vi "set range property lecroy.vi"(0 "VISA in":refnum<visa-resource-name>, 5 "Group":string, 7 "Property":T1, 9 "Value":variant, 11 "error in":errorcluster, 12 "First Channel":T2={" Card.Channel"=1.12, "Crate"=0} {"Card.Channel" format="%.2f"}, 13 "Num Channels":i32) -> (4 "VISA out":refnum<visa-resource-name>, 15 "error out":errorcluster)   [LabVIEW 2018]
uses:
  channel.ctl
  Group Properties.ctl
  Tom Shaw/Lecroy Control/HV Documentation and Software for Testing/SubVIs/General_lecroy_command.ctl
  CAEN globals.vi
  <vilib>/regexp/Match Regular Expression.xnode
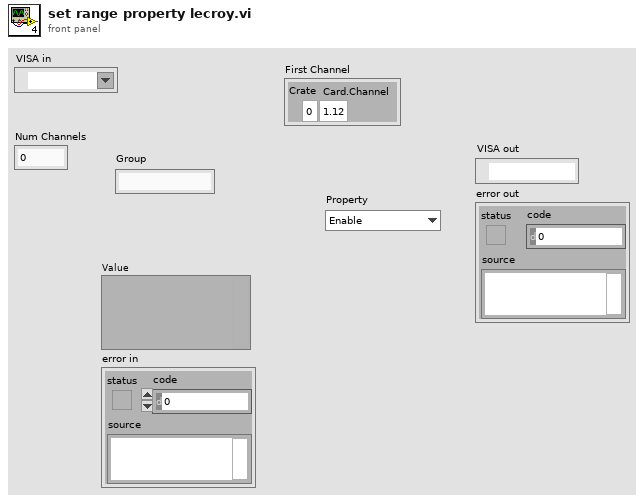
[diagram p1: front panel]
types:
  T1 = typedef "Group Properties.ctl" = enum16{"Enable", "Vset", "Imax", "Vswmax", "Trip Time"}
  T2 = typedef "channel.ctl" = cluster{" Card.Channel":dbl, "Crate":i32}
  T3 = enum16{"Monitor", "Demand", "Backup", "All", "None"}
  T4 = typedef "General_lecroy_command.ctl" = string
  T5 = typedef "channel_cluster.ctl" = cluster{"Channel Name":string, "Crate":i32, "Card Type":string, "Card":i32, "Channel":i32, "Status Icon":picture, "Vmon (V)":dbl, "Vset (V)":dbl, "Imon (A)":dbl, "Iset (A)":dbl, "Timestamp":string, "ON/OFF":bool, "Status":string, "Vswmax (V)":dbl, "Flag":bool, "Vfile (V)":dbl, "Error Logged":bool[], "enable_file":bool}
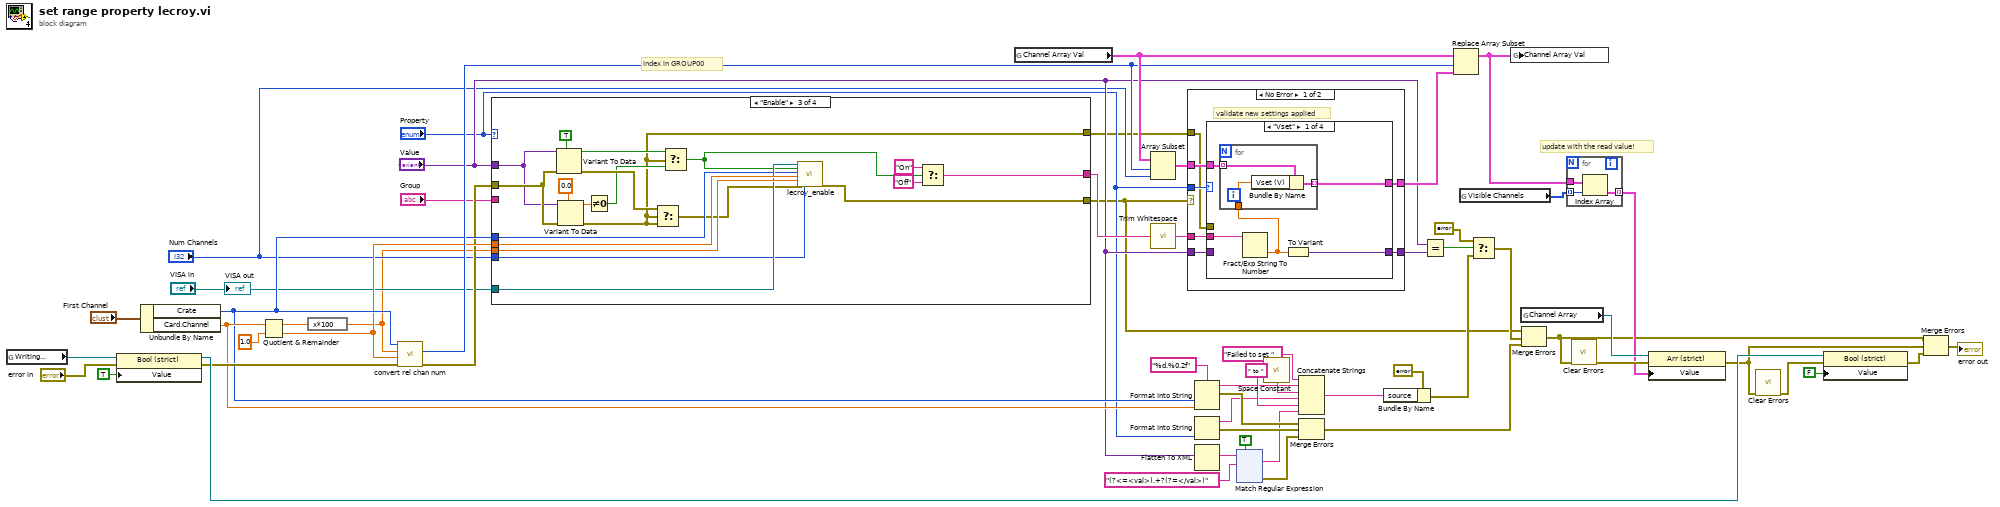
[diagram p0: block diagram]
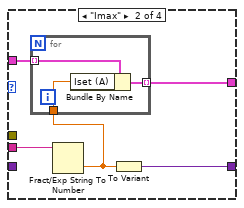
[diagram p2: hidden frame]
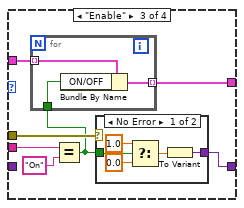
[diagram p3: hidden frame]
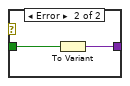
[diagram p4: hidden frame]
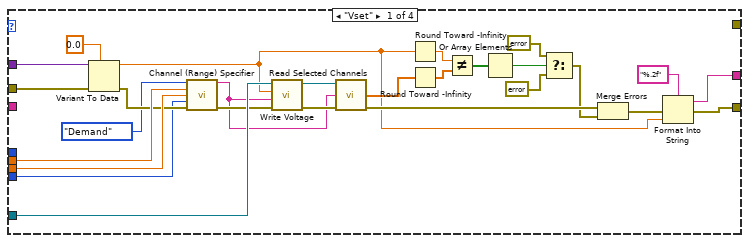
[diagram p7: hidden frame]
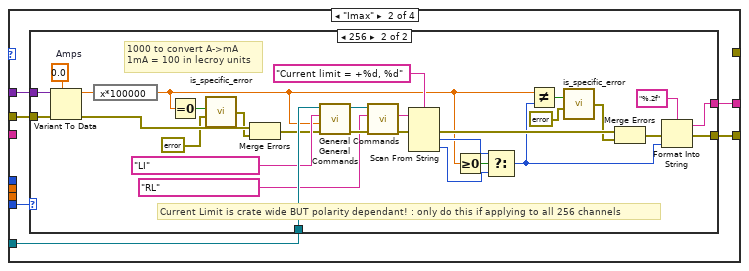
[diagram p8: hidden frame]
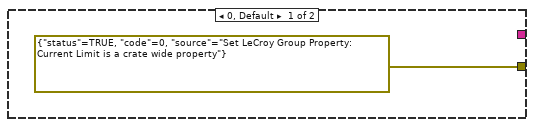
[diagram p9: hidden frame]
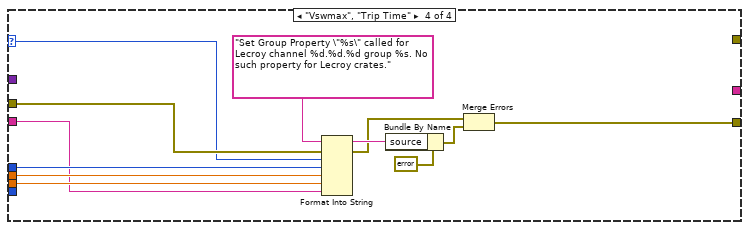
[diagram p10: hidden frame]
diagram:
  # "index in GROUP00"
  # "update with the read value!"
  n1 = global read "CAEN globals.vi" "Writing..."() -> (w55:refnum<vi>)
  n2 = property class="Bool (strict)"(reference=w55, error in="error in", "Value"=TRUE) -> (reference out=w52:refnum<vi>, error out=w19:errorcluster)
  n3 = Unbundle By Name("First Channel") -> ("Crate"=w17:i32, "Card.Channel"=w18:dbl)
  n4 = Quotient & Remainder(x=w18, y=1.0) -> (x-y*floor(x/y)=w8:dbl, floor(x/y)=w16:dbl)
  n5 = expression code="x*100"(w8) -> (w7:dbl)
  n6 = call "convert rel chan num.vi"("error in"=w19, "Card"=w16, "Channel"=w7, "Crate"=w17) -> ("error out"=w14:errorcluster, "Absolute index"=w20:i32)  [unwired: 4 in, 2 out]
  n7 = case shown="\"Enable\"" "Property" {
    selector: "Property" -> [_ _ _ w146]
    tunnel: [w72 w88 w137 _] -> w15
    tunnel: "Value" -> [w84 w91 w131 _]
    tunnel: [w73 w89 w138 w150] -> w6
    tunnel: w14 -> [w83 w90 w132 w153]
    tunnel: w17 -> [_ _ w139 w147]
    tunnel: "VISA in" -> [w82 w87 w140 _]
    tunnel: w7 -> [w80 _ w142 w144]
    tunnel: w16 -> [w81 _ w141 w145]
    tunnel: "Num Channels" -> [w63 w86 w124 _]
    tunnel: "Group" -> [_ _ _ w143]
    tunnel: [_ _ w123 _] -> w4
    frame "Vset" {
      n8 = Variant To Data(error in=w83, type=0.0 ("precision (6)"), Variant=w84) -> (data=w59:dbl, error out=w79:errorcluster)
      n9 = call "Channel (Range) Specifier.vi"("Buffer"=T3."Demand", "Card"=w81, "Channel"=w80, "Num Channels"=w63, "error in"=w79) -> ("Channel (Range)"=w75:string, "error out"=w78:errorcluster)  [unwired: 9 in]
      n10 = call "Write Voltage.vi"("error in"=w78, "Channel+Range"=w75, "Voltage input"=w59, "VISA in"=w82) -> ("error out"=w76:errorcluster, "VISA out"=w74:refnum<visa-resource-name>)  [unwired: 5 in, 1 out]
      n11 = call "Read Selected Channels.vi"("VISA in"=w74, "C##,##DO###"=w75, "error in"=w76) -> ("Selected Buffer"=w62:dbl[], "error out"=w66:errorcluster)  [unwired: 6 in, 5 out]
      n12 = Round Toward -Infinity(1:w59) -> (0:w70:dbl)
      n13 = Round Toward -Infinity(1:w62) -> (0:w69:dbl[])
      n14 = Not Equal?(x=w70, y=w69) -> (x != y?=w61:bool[])
      n15 = Or Array Elements(Boolean array=w61) -> (logical OR=w60:bool)
      n16 = Select(t=errorcluster {"status"=TRUE, "code"=0, "source"="LeCroy Group Vset validation error"} ("error out"), s=w60, f=errorcluster {"status"=FALSE, "code"=0, "source"=""} ("error out")) -> (s? t:f=w65:errorcluster)
      n17 = Merge Errors(w66, w65) -> (w64:errorcluster)
      n18 = Format Into String(format string="%.2f", error in=w64, w59) -> (resulting string=w72:string, error out=w73:errorcluster)  [unwired: 1 in]
    }
    frame "Imax" {
      n19 = case shown="256" w86 {
        tunnel: w91 -> [_ w122]
        tunnel: w90 -> [_ w121]
        tunnel: [errorcluster {"status"=TRUE, "code"=0, "source"="Set LeCroy Group Property: Current Limit is a crate wide property"} ("error IO") w120] -> w89
        tunnel: [_ w119] -> w88
        tunnel: w87 -> [_ w118]
        frame 0, Default {
        }
        frame 256 {
          w117 = 0.0  # Amps
          # "Current Limit is crate wide BUT polarity dependant! : only do this if applying to all 256 channels"
          # "1000 to convert A->mA\n1mA = 100 in lecroy units"
          n20 = Variant To Data(error in=w121, type=w117, Variant=w122) -> (data=w110:dbl, error out=w99:errorcluster)
          n21 = expression code="x*100000"(w110) -> (w101:dbl)
          n22 = Equal To 0?(x=w101) -> (x = 0?=w100:bool)
          n23 = call "is_specific_error.vi"("Boolean"=w100, "error in (no error)"=errorcluster {"status"=TRUE, "code"=0, "source"="Request to set current limit to 0mA"} ("error out")) -> ("error out"=w94:errorcluster)  [unwired: 6 in]
          n24 = Merge Errors(w99, w94) -> (w98:errorcluster)
          n25 = call "General Commands.vi"("error in"=w98, "Current Limit"=w101, "Action"=T4 "LI", "VISA in"=w118) -> ("error out"=w113:errorcluster, "VISA out"=w114:refnum<visa-resource-name>)  [unwired: 5 in, 1 out]
          n26 = call "General Commands.vi"("error in"=w113, "Action"=T4 "RL", "VISA in"=w114) -> ("error out"=w108:errorcluster, "result string"=w106:string)  [unwired: 6 in, 1 out]
          n27 = Scan From String(format string="Current limit = +%d, %d", input string=w106, error in=w108) -> (error out=w107:errorcluster, output 1=w104:i32, output 2=w103:i32)  [unwired: 3 in, 2 out]
          n28 = Greater Or Equal To 0?(x=w101) -> (x >= 0?=w105:bool)
          n29 = Select(t=w104, s=w105, f=w103) -> (s? t:f=w102:i32)
          n30 = Not Equal?(x=w101, y=w102) -> (x != y?=w96:bool)
          n31 = call "is_specific_error.vi"("Boolean"=w96, "error in (no error)"=errorcluster {"status"=TRUE, "code"=0, "source"="LeCroy Group Vset validation error"} ("error out")) -> ("error out"=w97:errorcluster)  [unwired: 6 in]
          n32 = Merge Errors(w107, w97) -> (w115:errorcluster)
          n33 = Format Into String(format string="%.2f", error in=w115, w102) -> (resulting string=w119:string, error out=w120:errorcluster)  [unwired: 1 in]
        }
      }
    }
    frame "Enable" {
      n34 = Variant To Data(error in=w132, type=TRUE ("status"), Variant=w131) -> (data=w127:bool, error out=w130:errorcluster)
      n35 = Variant To Data(error in=w132, type=0.0, Variant=w131) -> (data=w129:dbl, error out=w123:errorcluster)
      n36 = Not Equal To 0?(x=w129) -> (x != 0?=w128:bool)
      n37 = Select(t=w130, s=w123, f=w123) -> (s? t:f=w125:errorcluster)
      n38 = Select(t=w127, s=w123, f=w128) -> (s? t:f=w126:bool)
      n39 = call "lecroy_enable.vi"("VISA in"=w140, "Enable"=w126, "Crate"=w139, "Card"=w141, "Channel"=w142, "error in"=w125, "Num Channels"=w124) -> ("error out"=w138:errorcluster)  [unwired: 10 in, 2 out]
      n40 = Select(t="On" ("format string"), s=w126, f="Off" ("format string")) -> (s? t:f=w137:string)
    }
    frame "Vswmax", "Trip Time" {
      n41 = Format Into String(format string="Set Group Property \"%s\" called for Lecroy channel %d.%d.%d group %s. No such property for Lecroy crates." ("source"), error in=w153, w146, w147, w145, w144, w143) -> (resulting string=w151:string, error out=w148:errorcluster)  [unwired: 1 in]
      n42 = Bundle By Name(cluster=errorcluster {"status"=TRUE, "code"=0, "source"=""} ("error out"), "source"=w151) -> (w149:errorcluster)
      n43 = Merge Errors(w148, w149) -> (w150:errorcluster)
    }
  }
  n44 = global read "CAEN globals.vi" "Channel Array Val"() -> (w45:T5[])
  n45 = Array Subset(array=w45, index=w20, length="Num Channels") -> (w48:T5[])
  n46 = call <vilib>:"Trim Whitespace.vi"("string"=w15) -> ("trimmed string"=w49:string)  [unwired: 1 in]
  n47 = case shown="No Error" w6 {
    tunnel: [w161 w198] -> w58
    tunnel: w49 -> [w160 _]
    tunnel: w48 -> [w159 w197]
    tunnel: [w158 w197] -> w46
    tunnel: "Property" -> [w157 _]
    tunnel: "Value" -> [w156 w198]
    tunnel: w4 -> [w155 _]
    frame No Error {
      # "validate new settings applied"
      n48 = case shown="\"Vset\"" w157 {
        tunnel: w160 -> [w165 w173 w183 _]
        tunnel: [w166 w174 w184 w195] -> w161
        tunnel: w159 -> [w164 w172 w181 w196]
        tunnel: [w162 w170 w180 w196] -> w158
        tunnel: w156 -> [_ _ _ w195]
        tunnel: w155 -> [_ _ w179 _]
        frame "Vset" {
          n49 = Fract/Exp String To Number(string=w165) -> (number=w163:dbl)  [unwired: 3 in, 1 out]
          n50 = for {
            tunnel: w164 -> [w169] mode=indexing
            tunnel: w163 -> [w168]
            tunnel: [w167] -> w162 mode=indexing
            n51 = Bundle By Name(cluster=w169, "Vset (V)"=w168) -> (w167:T5)
          }
          n52 = To Variant(anything=w163) -> (Variant=w166:variant)
        }
        frame "Imax" {
          n53 = Fract/Exp String To Number(string=w173) -> (number=w171:dbl)  [unwired: 3 in, 1 out]
          n54 = for {
            tunnel: w172 -> [w177] mode=indexing
            tunnel: w171 -> [w176]
            tunnel: [w175] -> w170 mode=indexing
            n55 = Bundle By Name(cluster=w177, "Iset (A)"=w176) -> (w175:T5)
          }
          n56 = To Variant(anything=w171) -> (Variant=w174:variant)
        }
        frame "Enable" {
          n57 = Equal?(x=w183, y="On" ("x")) -> (x = y?=w178:bool)
          n58 = for {
            tunnel: w181 -> [w194] mode=indexing
            tunnel: [w193] -> w180 mode=indexing
            tunnel: w178 -> [w192]
            n59 = Bundle By Name(cluster=w194, "ON/OFF"=w192) -> (w193:T5)
          }
          n60 = case shown="No Error" w179 {
            tunnel: [w189 w191] -> w184
            tunnel: w178 -> [w187 w190]
            frame No Error {
              n61 = Select(t=1.0, s=w187, f=0.0) -> (s? t:f=w188:dbl)
              n62 = To Variant(anything=w188) -> (Variant=w189:variant)
            }
            frame Error {
              n63 = To Variant(anything=w190) -> (Variant=w191:variant)
            }
          }
        }
        frame "Vswmax", "Trip Time" {
        }
      }
    }
    frame Error {
    }
  }
  n64 = Format Into String(format string="%d.%0.2f", w17, w18) -> (resulting string=w33:string, error out=w30:errorcluster)  [unwired: 2 in]
  n65 = Format Into String("Property") -> (resulting string=w28:string, error out=w29:errorcluster)  [unwired: 3 in]
  n66 = Flatten To XML(anything="Value") -> (xml string=w27:string)
  n67 = xnode "Match Regular Expression"("input string"=w27, "regular expression"="(?<=<val>).+?(?=</val>)" ("xml string"), "ignore case? (F)"=TRUE) -> ("whole match"=w24:string, "error out"=w23:errorcluster)  [unwired: 3 in, 3 out]
  n68 = call <vilib>:"Space Constant.vi"() -> ("String"=w37:string)
  n69 = Concatenate Strings("Failed to set " ("source"), w33, w37, w28, " to " ("string"), w24) -> (w39:string)
  n70 = Merge Errors(w30, w29, w23) -> (w31:errorcluster)
  n71 = Bundle By Name(cluster=errorcluster {"status"=TRUE, "code"=0, "source"="Value not set"} ("error in"), "source"=w39) -> (w34:errorcluster)
  n72 = Equal?(x="Value", y=w58) -> (x = y?=w57:bool)
  n73 = Replace Array Subset(array=w45, new element=w46, index=w20) -> (w44:T5[])
  n74 = global read "CAEN globals.vi" "Visible Channels"() -> (w43:i32[])
  n75 = Select(t=errorcluster {"status"=FALSE, "code"=0, "source"=""} ("error in"), s=w57, f=w34) -> (s? t:f=w56:errorcluster)
  n76 = global write "CAEN globals.vi" "Channel Array Val"(w44) -> ()
  n77 = global read "CAEN globals.vi" "Channel Array"() -> (w42:refnum<vi>)
  n78 = Merge Errors(w6, w56, w31) -> (w3:errorcluster)
  n79 = for {
    tunnel: w44 -> [w201]
    tunnel: w43 -> [w200] mode=indexing
    tunnel: [w199] -> w41 mode=indexing
    n80 = Index Array(array=w201, index=w200) -> (element=w199:T5)
  }
  n81 = call <vilib>:"Clear Errors.vi"("error in (no error)"=w3) -> ("error out"=w47:errorcluster)  [unwired: 5 in, 1 out]
  n82 = property class="Arr (strict)"(reference=w42, error in=w47, "Value"=w41) -> (error out=w2:errorcluster)  [unwired: 1 out]
  n83 = call <vilib>:"Clear Errors.vi"("error in (no error)"=w2) -> ("error out"=w1:errorcluster)  [unwired: 5 in, 1 out]
  n84 = property class="Bool (strict)"(reference=w52, error in=w1, "Value"=FALSE) -> (error out=w51:errorcluster)  [unwired: 1 out]
  n85 = Merge Errors(w3, w2, w51) -> (→"error out":errorcluster)
  "VISA out" <- "VISA in"
